vi "Find Sift Proxy Binary.vi"(8 "error in (no error)":errorcluster, 11 "Sift Client in":refnum<class "Sift Client.lvclass">) -> (0 "error out":errorcluster, 1 "Found":bool, 2 "Path":path, 3 "Sift Client out":refnum<class "Sift Client.lvclass">)   [LabVIEW 2024, in "Sift Client.lvlib" / "Sift Client.lvclass"]
doc: "Finds the Sift Proxy binary (sift_proxy)."
uses:
  Sift Client.lvclass
  <vilib>/Utility/sysdir.llb/System Directory Type.ctl
  <vilib>/regexp/Match Regular Expression.xnode
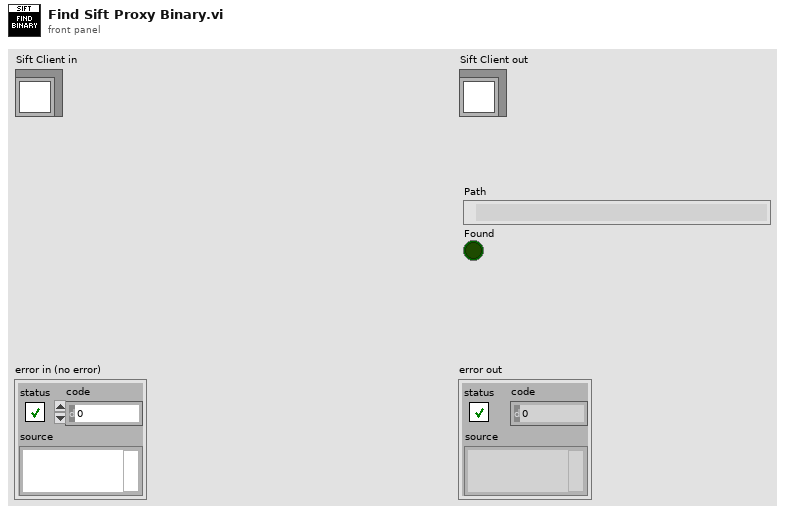
[diagram p1: front panel]
types:
  T1 = typedef "System Directory Type.ctl" = i32
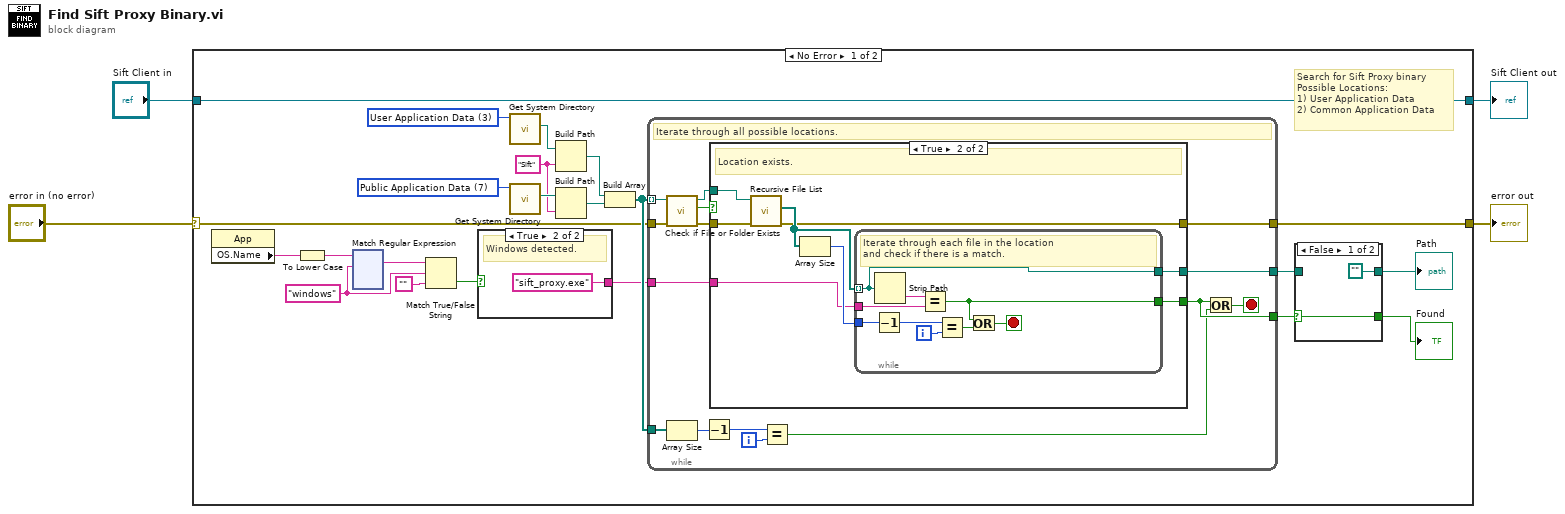
[diagram p0: block diagram]
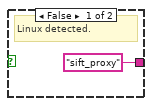
[diagram p2: hidden frame]
diagram:
  n1 = case shown="No Error" "error in (no error)" {
    selector: "error in (no error)" -> [w13 w185]
    tunnel: [w12 w185] -> w3
    tunnel: [w26 w184] -> w1
    tunnel: "Sift Client in" -> [w26 w184]
    frame No Error {
      w7 = "windows"
      w21 = "Sift"
      w23 = T1 7 items=["User Home"=0, "User Desktop"=1, "User Documents"=2, "User Application Data"=3, "User Preferences"=4, "User Temporary"=5, "Public Documents"=6, "Public Application Data"=7, "Public Preferences"=8, "Public Cache"=13, "System Core Libraries"=9, "System Installed Libraries"=10, "Application Files"=11, "Boot Volume Root"=12] ("system directory type")
      w25 = T1 3 items=["User Home"=0, "User Desktop"=1, "User Documents"=2, "User Application Data"=3, "User Preferences"=4, "User Temporary"=5, "Public Documents"=6, "Public Application Data"=7, "Public Preferences"=8, "Public Cache"=13, "System Core Libraries"=9, "System Installed Libraries"=10, "Application Files"=11, "Boot Volume Root"=12] ("system directory type")
      # "Search for Sift Proxy binary\nPossible Locations:\n1) User Application Data\n2) Common Application Data"
      n2 = property class="App"() -> ("OS.Name"=w11:string)  [unwired: 2 in, 2 out]
      n3 = To Lower Case(string=w11) -> (all lower case string=w10:string)
      n4 = xnode "Match Regular Expression"("input string"=w10, "regular expression"=w7) -> ("whole match"=w9:string)  [unwired: 4 in, 4 out]
      n5 = Match True/False String(2:"", 3:w7, 4:w9) -> (0:w6:bool)  [unwired: 1 out]
      n6 = case shown="True" w6 {
        tunnel: ["sift_proxy" "sift_proxy.exe"] -> w5
        frame False {
          # "Linux detected."
        }
        frame True {
          # "Windows detected."
        }
      }
      n7 = call <vilib>:"Get System Directory.vi"("system directory type"=w25) -> ("system directory"=w24:path)  [unwired: 10 in]
      n8 = call <vilib>:"Get System Directory.vi"("system directory type"=w23) -> ("system directory"=w22:path)  [unwired: 10 in]
      n9 = Build Path(base path=w24, name or relative path=w21) -> (appended path=w20:path)
      n10 = Build Path(base path=w22, name or relative path=w21) -> (appended path=w19:path)
      n11 = Build Array(w20, w19) -> (w14:path[])
      n12 = while {
        tunnel: w14 -> [w158] mode=indexing
        tunnel: [w160] -> w17
        tunnel: [w156] -> w15
        tunnel: w14 -> [w154]
        tunnel: w13 -> [w149]
        tunnel: [w147] -> w12
        tunnel: w5 -> [w146]
        i -> [w151]
        stop <- w155 stop-if-true
        # "Iterate through all possible locations."
        n13 = call <vilib>:"Check if File or Folder Exists.vi"("error in (no error)"=w149, "path"=w158) -> ("error out"=w148:errorcluster, "file or folder exists?"=w159:bool, "dup path"=w157:path)  [unwired: 7 in]
        n14 = Array Size(array=w154) -> (size(s)=w153:i32)
        n15 = Decrement(x=w153) -> (x-1=w152:i32)
        n16 = case shown="True" w159 {
          selector: w159 -> [w162 _]
          tunnel: w157 -> [_ w170]
          tunnel: [_ w167] -> w160
          tunnel: [w162 w166] -> w156
          tunnel: w148 -> [w161 w165]
          tunnel: [w161 w164] -> w147
          tunnel: w146 -> [_ w163]
          frame False {
            # "Location does not exist."
          }
          frame True {
            # "Location exists."
            n17 = call <vilib>:"Recursive File List.vi"("error in (no error)"=w165, "Folder Path"=w170) -> ("error out"=w164:errorcluster, "All Files in Dir"=w169:path[])  [unwired: 5 in, 3 out]
            n18 = Array Size(array=w169) -> (size(s)=w168:i32)
            n19 = while {
              tunnel: w169 -> [w174] mode=indexing
              tunnel: w168 -> [w177]
              tunnel: [w174] -> w167
              tunnel: [w171] -> w166
              tunnel: w163 -> [w172]
              i -> [w178]
              stop <- w175 stop-if-true
              # "Iterate through each file in the location \nand check if there is a match."
              n20 = Decrement(x=w177) -> (x-1=w176:i32)
              n21 = Strip Path(path=w174) -> (name=w173:string)  [unwired: 1 out]
              n22 = Equal?(x=w173, y=w172) -> (x = y?=w171:bool)
              n23 = Equal?(x=w176, y=w178) -> (x = y?=w179:bool)
              n24 = Or(x=w171, y=w179) -> (x .or. y?=w175:bool)
            }
          }
        }
        n25 = Equal?(x=w152, y=w151) -> (x = y?=w150:bool)
        n26 = Or(x=w156, y=w150) -> (x .or. y?=w155:bool)
      }
      n27 = case shown="False" w15 {
        selector: w15 -> [w181 w182]
        tunnel: [path "" w183] -> w18
        tunnel: w17 -> [_ w183]
        tunnel: [w181 w182] -> w16
        frame False {
        }
        frame True {
        }
      }
      "Path" <- w18
      "Found" <- w16
    }
    frame Error {
    }
  }
  "error out" <- w3
  "Sift Client out" <- w1
